vi "UtilityLib.get unused TCP port.vi"(2 "TCP port offset":u16, 5 "error in (no error)":errorcluster) -> (16 "TCP port":u16, 19 "error out":errorcluster)   [LabVIEW 2014, in "UtilityLib.lvlib"]
doc: "Obtains an unsed TCP port on the local machine."
uses:
  UtilityLib.lvlib
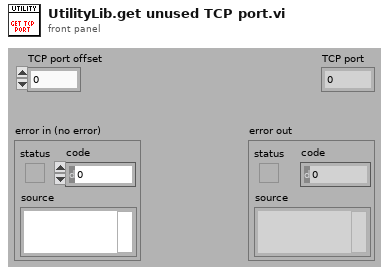
[diagram p1: front panel]
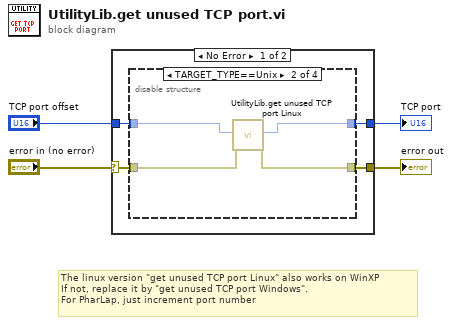
[diagram p0: block diagram]
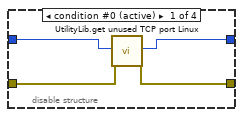
[diagram p2: hidden frame]
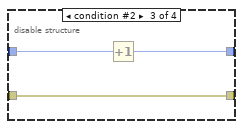
[diagram p3: hidden frame]
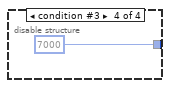
[diagram p4: hidden frame]
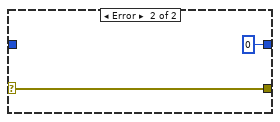
[diagram p5: hidden frame]
diagram:
  # "The linux version \"get unused TCP port Linux\" also works on WinXP\nIf not, replace it by \"get unused TCP port Windows\".\nFor PharLap, just increment port number"
  n1 = case shown="No Error" "error in (no error)" {
    selector: "error in (no error)" -> [w5 w22]
    tunnel: "TCP port offset" -> [w8 _]
    tunnel: [w7 w22] -> w3
    tunnel: [w6 u16 0 ("TCP port")] -> w2
    frame No Error {
      n2 = disable-structure "Conditional Disable Structure" shown="TARGET_TYPE==Unix" {
        disable-tunnel: w8 -> [w12 w16 w19 _]
        disable-tunnel: w5 -> [w11 w15 w18 _]
        disable-tunnel: [w10 w14 w18 _] -> w7
        disable-tunnel: [w9 w13 w17 u16 7000 ("TCP port")] -> w6
        frame condition #0 (active) {
          n3 = call "UtilityLib.get unused TCP port Linux.vi"("TCP port offset"=w12, "error in (no error)"=w11) -> ("TCP port"=w9:u16, "error out"=w10:errorcluster)  [unwired: 16 in]
        }
        frame condition #1 {
          n4 = call "UtilityLib.get unused TCP port Linux.vi"("TCP port offset"=w16, "error in (no error)"=w15) -> ("TCP port"=w13:u16, "error out"=w14:errorcluster)  [unwired: 16 in]
        }
        frame condition #2 {
          n5 = Increment(x=w19) -> (x+1=w17:u16)
        }
        frame condition #3 {
        }
      }
    }
    frame Error {
    }
  }
  "TCP port" <- w2
  "error out" <- w3
